vi "f2f (SubVI).vi"(2 "ptFrame2":T2[](array[typedef]), 3 "ptFrame1":T2[](array[typedef]), 4 "InverseA":T1) -> (0 "CoMxyz":dbl[](array[numeric]), 1 "xyzpyr":dbl[](array[numeric]))   [LabVIEW 2021]
uses:
  ctrOWLMarker.ctl
  <vilib>/Analysis/Matrix/Datatypes/RealMatrix.ctl
  <vilib>/Analysis/coordinate.llb/Euler Rotation Order.ctl
  <vilib>/Analysis/baseanly.llb/Real A x B.vi
  <vilib>/Analysis/baseanly.llb/Mean (DBL).vi
  <vilib>/Analysis/Matrix/Numeric/Conversions/Array To Matrix - RA.vi
  <vilib>/Analysis/Matrix/Numeric/Conversions/Matrix To Array - RM.vi
  <vilib>/Analysis/Matrix/NI_Matrix.lvlib
  <vilib>/Analysis/NI_AALBase.lvlib
  <vilib>/Analysis/NI_AALPro.lvlib
panel:
  out "Euler Angles":cluster{"phi":dbl, "theta":dbl, "psi":dbl}
  out "translationXYZ":dbl[](array[numeric])
  out "Rmatrix":T1
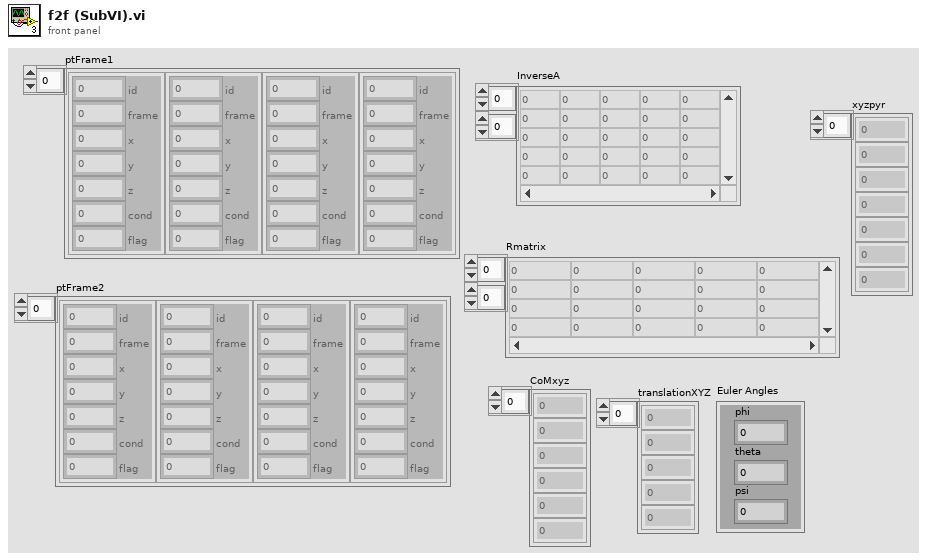
[diagram p1: front panel]
types:
  T1 = typedef "NI_Matrix.lvlib/RealMatrix.ctl" = dbl[][]
  T2 = typedef "ctrOWLMarker.ctl" = cluster{"id":i32, "frame":i32, "x":sgl, "y":sgl, "z":sgl, "cond":sgl, "flag":u32}
  T3 = typedef "NI_AALPro.lvlib/Euler Rotation Order.ctl" = u16
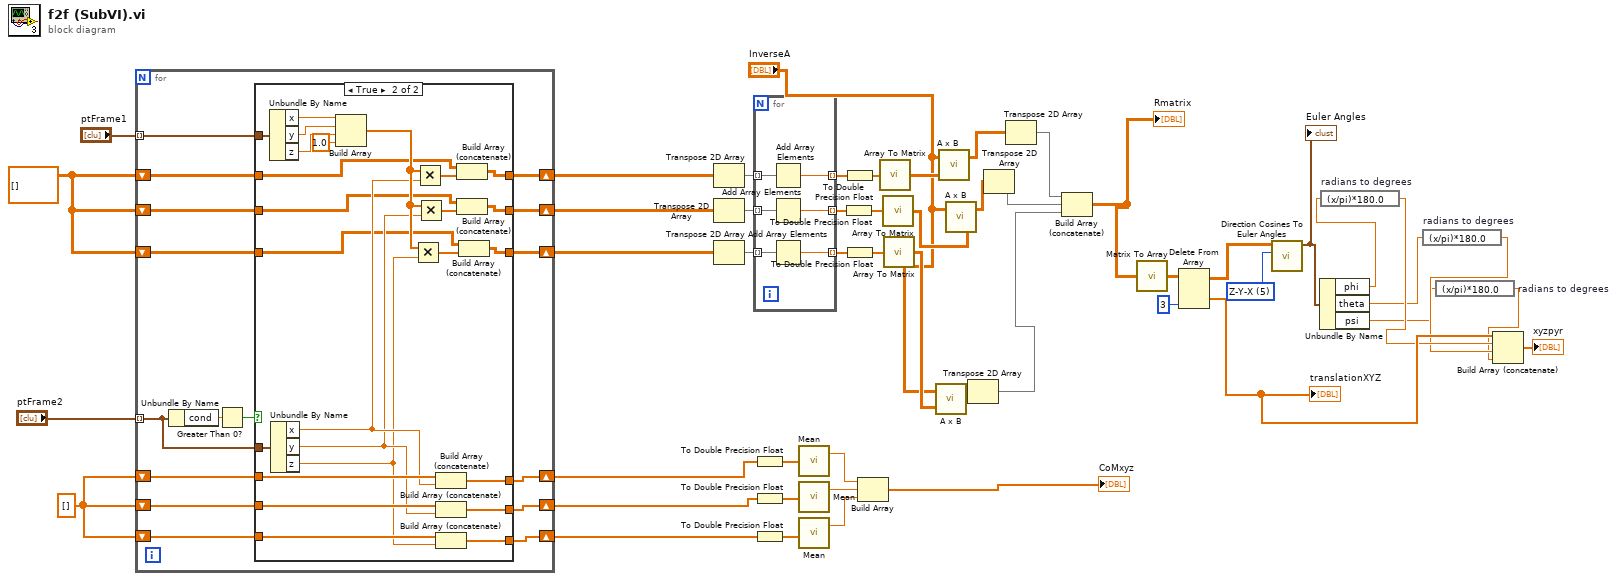
[diagram p0: block diagram]
diagram:
  w10 = T3 5 items=["X-Y-Z", "X-Z-Y", "Y-X-Z", "Y-Z-X", "Z-X-Y", "Z-Y-X", "X-Y-X", "X-Z-X", "Y-X-Y", "Y-Z-Y", "Z-X-Z", "Z-Y-Z"] ("rotation order")
  w38 = sgl[][] []
  w39 = sgl[] []
  n1 = for {
    tunnel: "ptFrame2" -> [w65] mode=indexing
    shift-right: [w63] -> w50
    shift-left: w39 -> [w64]
    shift-right: [w61] -> w43
    shift-left: w39 -> [w60]
    shift-right: [w62] -> w42
    shift-left: w39 -> [w59]
    tunnel: "ptFrame1" -> [w57] mode=indexing
    shift-right: [w56] -> w37
    shift-left: w38 -> [w53]
    shift-right: [w55] -> w34
    shift-left: w38 -> [w52]
    shift-right: [w54] -> w35
    shift-left: w38 -> [w51]
    n2 = Unbundle By Name(w65) -> ("cond"=w66:sgl)
    n3 = Greater Than 0?(x=w66) -> (x > 0?=w58:bool)
    n4 = case shown="True" w58 {
      tunnel: w65 -> [_ w97]
      tunnel: w64 -> [w72 w96]
      tunnel: [w72 w95] -> w63
      tunnel: [w70 w94] -> w62
      tunnel: [w71 w93] -> w61
      tunnel: w60 -> [w71 w92]
      tunnel: w59 -> [w70 w91]
      tunnel: w57 -> [_ w90]
      tunnel: [w69 w78] -> w56
      tunnel: [w68 w77] -> w55
      tunnel: [w67 w76] -> w54
      tunnel: w53 -> [w69 w75]
      tunnel: w52 -> [w68 w74]
      tunnel: w51 -> [w67 w73]
      frame False {
      }
      frame True {
        n5 = Unbundle By Name(w90) -> ("x"=w89:sgl, "y"=w88:sgl, "z"=w87:sgl)
        n6 = Unbundle By Name(w97) -> ("x"=w84:sgl, "y"=w83:sgl, "z"=w82:sgl)
        n7 = Build Array(w89, w88, w87, sgl 1.0 ("element")) -> (w85:sgl[])
        n8 = Multiply(x=w85, y=w82) -> (x*y=w79:sgl[])
        n9 = Multiply(x=w85, y=w84) -> (x*y=w81:sgl[])
        n10 = Multiply(x=w85, y=w83) -> (x*y=w80:sgl[])
        n11 = Build Array (concatenate)(w96, w84) -> (w95:sgl[])
        n12 = Build Array (concatenate)(w92, w83) -> (w93:sgl[])
        n13 = Build Array (concatenate)(w91, w82) -> (w94:sgl[])
        n14 = Build Array (concatenate)(w75, w81) -> (w78:sgl[][])
        n15 = Build Array (concatenate)(w74, w80) -> (w77:sgl[][])
        n16 = Build Array (concatenate)(w73, w79) -> (w76:sgl[][])
      }
    }
  }
  n17 = Transpose 2D Array(2D array=w37) -> (transposed array=w36:sgl[][])
  n18 = Transpose 2D Array(2D array=w34) -> (transposed array=w33:sgl[][])
  n19 = Transpose 2D Array(2D array=w35) -> (transposed array=w32:sgl[][])
  n20 = for {
    tunnel: w36 -> [w98] mode=indexing
    tunnel: w33 -> [w103] mode=indexing
    tunnel: w32 -> [w102] mode=indexing
    tunnel: [w101] -> w31 mode=indexing
    tunnel: [w100] -> w30 mode=indexing
    tunnel: [w99] -> w29 mode=indexing
    n21 = Add Array Elements(numeric array=w98) -> (sum=w101:sgl)
    n22 = Add Array Elements(numeric array=w103) -> (sum=w100:sgl)
    n23 = Add Array Elements(numeric array=w102) -> (sum=w99:sgl)
  }
  n24 = To Double Precision Float(number=w50) -> (double precision float=w49:dbl[])
  n25 = To Double Precision Float(number=w43) -> (double precision float=w48:dbl[])
  n26 = To Double Precision Float(number=w42) -> (double precision float=w47:dbl[])
  n27 = call-poly <vilib>:"Mean.vi"("X"=w49) -> ("mean"=w46:dbl)  [unwired: 1 out]
  n28 = call-poly <vilib>:"Mean.vi"("X"=w48) -> ("mean"=w45:dbl)  [unwired: 1 out]
  n29 = call-poly <vilib>:"Mean.vi"("X"=w47) -> ("mean"=w44:dbl)  [unwired: 1 out]
  n30 = To Double Precision Float(number=w30) -> (double precision float=w27:dbl[])
  n31 = To Double Precision Float(number=w31) -> (double precision float=w18:dbl[])
  n32 = To Double Precision Float(number=w29) -> (double precision float=w28:dbl[])
  n33 = Build Array(w46, w45, w44) -> (→"CoMxyz":dbl[])
  n34 = call-poly <vilib>:"Array To Matrix.vi"("Real 1D Array"=w18) -> ("Real Matrix (Column Vector)"=w24:T1)
  n35 = call-poly <vilib>:"Array To Matrix.vi"("Real 1D Array"=w27) -> ("Real Matrix (Column Vector)"=w25:T1)
  n36 = call-poly <vilib>:"Array To Matrix.vi"("Real 1D Array"=w28) -> ("Real Matrix (Column Vector)"=w26:T1)
  n37 = call-poly <vilib>:"A x B.vi"("B"=w26, "A"="InverseA") -> ("A x B"=w21:T1)  [unwired: 1 out]
  n38 = call-poly <vilib>:"A x B.vi"("B"=w24, "A"="InverseA") -> ("A x B"=w23:T1)  [unwired: 1 out]
  n39 = call-poly <vilib>:"A x B.vi"("B"=w25, "A"="InverseA") -> ("A x B"=w22:T1)  [unwired: 1 out]
  n40 = Transpose 2D Array(2D array=w21) -> (transposed array=w15:T1)
  n41 = Transpose 2D Array(2D array=w22) -> (transposed array=w16:T1)
  n42 = Transpose 2D Array(2D array=w23) -> (transposed array=w17:T1)
  n43 = Build Array (concatenate)(w17, w16, w15) -> (w14:T1)
  "Rmatrix" <- w14
  n44 = call-poly <vilib>:"Matrix To Array.vi"("Real Matrix"=w14) -> ("Real 2D Array"=w11:dbl[][])
  n45 = Delete From Array(array=w11, index (col)=3 ("disabled index (col)")) -> (deleted portion=w8:dbl[], array with subset deleted=w12:dbl[][])  [unwired: 2 in]
  "translationXYZ" <- w8
  n46 = call <vilib>:"Direction Cosines To Euler Angles.vi"("rotation order"=w10, "Direction Cosines"=w12) -> ("Euler Angles"=w9:cluster{"phi":dbl, "theta":dbl, "psi":dbl})  [unwired: 8 in, 1 out]
  "Euler Angles" <- w9
  n47 = Unbundle By Name(w9) -> ("phi"=w6:dbl, "theta"=w4:dbl, "psi"=w2:dbl)
  n48 = expression code="(x/pi)*180.0" "radians to degrees"(w6) -> (w5:dbl)
  n49 = expression code="(x/pi)*180.0" "radians to degrees"(w4) -> (w3:dbl)
  n50 = expression code="(x/pi)*180.0" "radians to degrees"(w2) -> (w1:dbl)
  n51 = Build Array (concatenate)(w8, w5, w3, w1) -> (→"xyzpyr":dbl[])
